vi "Run.vi"(8 "error in (no error)":errorcluster, 10 "TestCase":refnum<class "TestCase.lvclass">, 11 "TestResult in":refnum<class "TestResult.lvclass">) -> (0 "error out":errorcluster, 2 "TestCase out":refnum<class "TestCase.lvclass">, 3 "TestResult out":refnum<class "TestResult.lvclass">)   [LabVIEW 2019, in "TestResult.lvclass"]
doc: "Runs a <B>TestCase</B>."
uses:
  TestResult.lvclass
  TestCase/TestCase/TestCase.lvclass
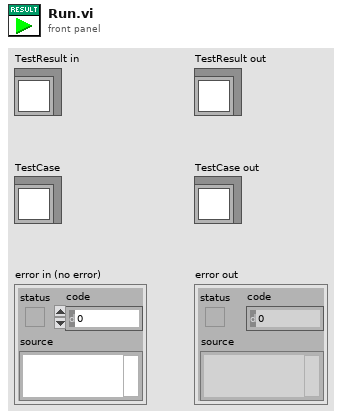
[diagram p1: front panel]
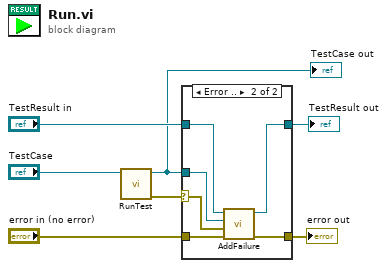
[diagram p0: block diagram]
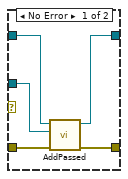
[diagram p2: hidden frame]
diagram:
  n1 = call-dynamic "RunTest.vi"("TestCase in"="TestCase") -> ("error out"=w6:errorcluster, "TestCase out"=w2:refnum<class "TestCase.lvclass">)  [unwired: 9 in]
  "TestCase out" <- w2
  n2 = case shown="Error .." w6 {
    selector: w6 -> [_ w18]
    tunnel: [w9 w14] -> w5
    tunnel: "TestResult in" -> [w10 w15]
    tunnel: "error in (no error)" -> [w12 w17]
    tunnel: w2 -> [w8 w16]
    tunnel: [w11 w13] -> w1
    frame No Error {
      n3 = call-dynamic "AddPassed.vi"("error in (no error)"=w12, "TestCase"=w8, "TestResult in"=w10) -> ("error out"=w11:errorcluster, "TestResult out"=w9:refnum<class "TestResult.lvclass">)  [unwired: 7 in]
    }
    frame Error {
      n4 = call-dynamic "AddFailure.vi"("error in (no error)"=w17, "Failure"=w18, "TestCase"=w16, "TestResult in"=w15) -> ("error out"=w13:errorcluster, "TestResult out"=w14:refnum<class "TestResult.lvclass">)  [unwired: 6 in]
    }
  }
  "error out" <- w1
  "TestResult out" <- w5
